vi "Create Folder.vi"(8 "error in (no error)":errorcluster, 10 "Strip File = T":bool, 11 "Path":path) -> (0 "error out":errorcluster)   [LabVIEW 2017]
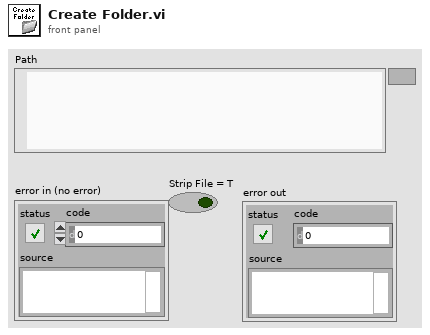
[diagram p1: front panel]
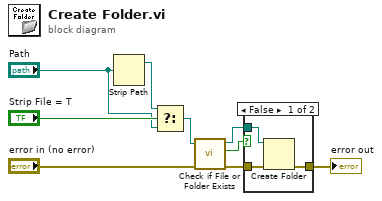
[diagram p0: block diagram]
diagram:
  n1 = Strip Path(path="Path") -> (stripped path=w4:path)  [unwired: 1 out]
  n2 = Select(t=w4, s="Strip File = T", f="Path") -> (s? t:f=w2:path)
  n3 = call <vilib>:"Check if File or Folder Exists.vi"("error in (no error)"="error in (no error)", "path"=w2) -> ("error out"=w7:errorcluster, "file or folder exists?"=w8:bool, "dup path"=w6:path)  [unwired: 7 in]
  n4 = case shown="False" w8 {
    tunnel: [w10 w13] -> w9
    tunnel: w7 -> [w11 w13]
    tunnel: w6 -> [w12 _]
    frame False {
      n5 = Create Folder(path (use dialog)=w12, error in=w11) -> (error out=w10:errorcluster)  [unwired: 1 in, 2 out]
    }
    frame True {
    }
  }
  "error out" <- w9
